vi "ExampleAsync.vi"() -> ()   [LabVIEW 2019, in "MicronTemplateAPIs.lvlib" / "MicronTemplateAPIs.lvclass"]
uses:
  MicronTemplateAPIs.lvclass
  vi.lib/Micron/gRPC/Client/Typedefs/AsyncMessageResponse.ctl
  vi.lib/Micron/gRPC/Client/Generated/MicronGRPCGeneratedClient/RPC Messages/micronGrpc_MessageRequest.ctl
  vi.lib/Micron/Base/Client/Typedefs/ServiceDetails.ctl
  78909296-a6b7-4131-b351-69347a1d12dc.vi
  9ceadd3c-745e-4cc0-becc-c9896ef65399.vi
  <vilib>/SLL Toolkit/SLL File IO/SLL File IO.lvlib
  vi.lib/Micron/Base/Client/MicronClient.lvclass
  vi.lib/Micron/gRPC/Client/Generated/MicronGRPCGeneratedClient/MicronGRPCGeneratedClient.lvlib
  vi.lib/Micron/gRPC/Client/MicronGRPCClient.lvclass
panel:
  in  "Collect Response?":bool
  out "Responses":T1[](array[typedef])
  in  "Repeat Count":i32=10
  in  "Connection Type":enum32{"Start New", "Connect Existing"}(tab)
  in  "Mode":string(combo)="Default"
  in  "Path":path
  in  "Port":i32=50051
  in  "ServiceID":string="micron-1"
  in  "UI":string(combo)="show"
  in  "Connection String":string="localhost:50051"
  out "error out":errorcluster
  in  "Command":string="Hello Micron!"
  in  "Payload":string="An Open Source Microservice Architecture on top of gRPC from https://github.com/KarthikAbiram/Micron"
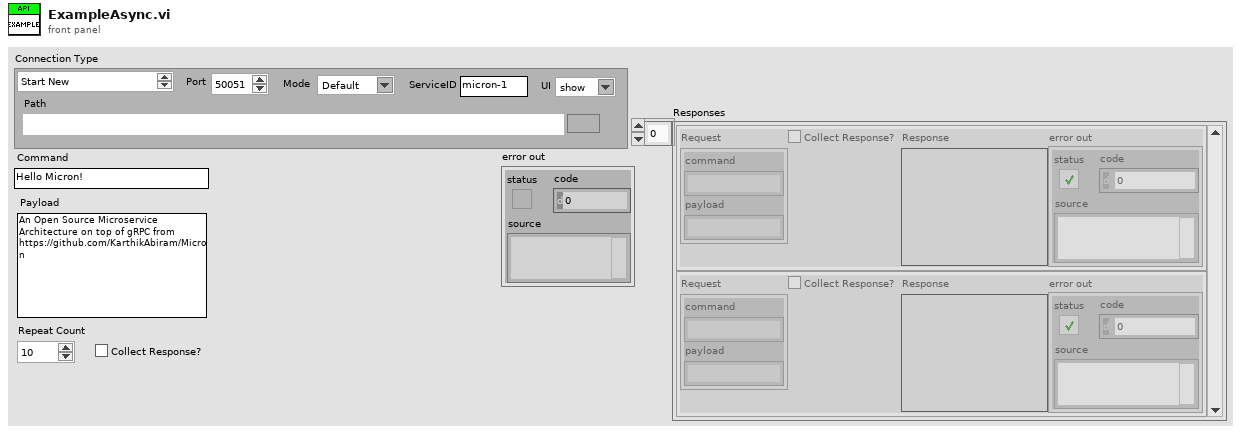
[diagram p1: front panel]
types:
  T1 = typedef "MicronGRPCClient.lvclass/AsyncMessageResponse.ctl" = cluster{"Request":T2, "Collect Response?":bool, "Response":string, "error out":errorcluster}
  T2 = typedef "MicronGRPCGeneratedClient.lvlib/micronGrpc_MessageRequest.ctl" = cluster{"command":string, "payload":string}
  T3 = typedef "MicronClient.lvclass/ServiceDetails.ctl" = cluster{"Micron Path":path, "Network":string, "ServiceID":string, "Port":i32, "FullyQualifiedName":string, "UI":string, "Args":string, "Mode":string}
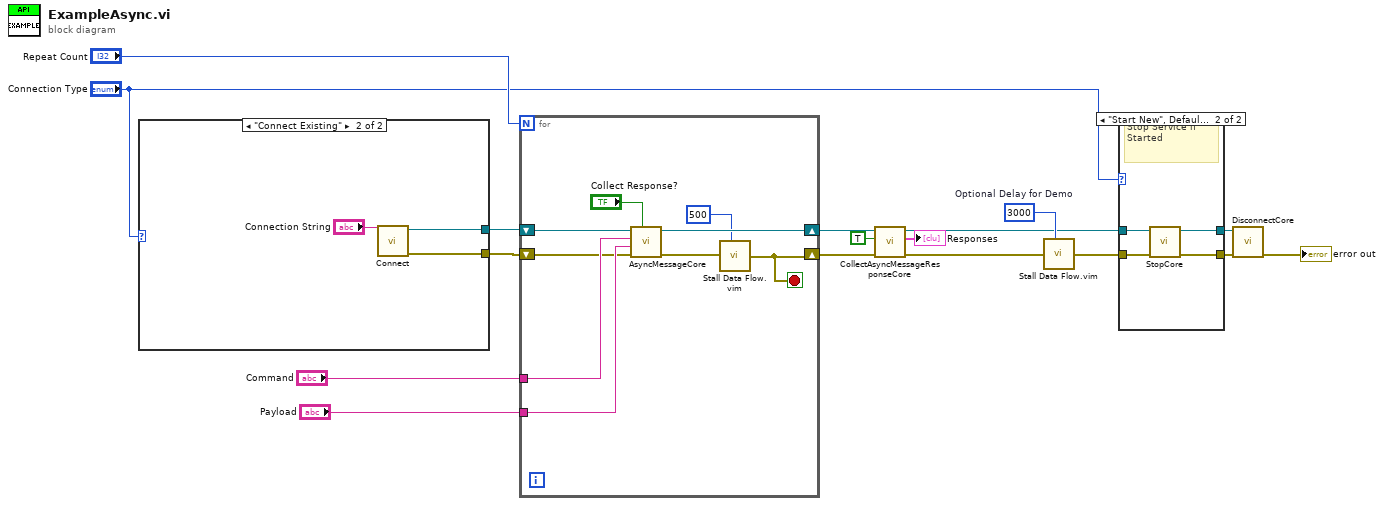
[diagram p0: block diagram]
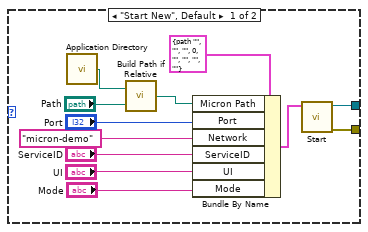
[diagram p3: hidden frame]
diagram:
  w9 = u32 3000  # Optional Delay for Demo
  n1 = case shown="\"Connect Existing\"" "Connection Type" {
    tunnel: [w29 w32] -> w14
    tunnel: [w28 w31] -> w13
    frame "Start New", Default {
      n2 = call <vilib>:"Application Directory.vi"() -> ("Application Directory"=w22:path)
      n3 = call <vilib>:"Build Path if Relative.vi"("Relative or Absolute Path"="Path", "Base Path"=w22) -> ("Path Out"=w23:path)
      n4 = Bundle By Name(cluster=T3 {"Micron Path"=path "", "Network"="", "ServiceID"="", "Port"=0, "FullyQualifiedName"="", "UI"="", "Args"="", "Mode"=""} ("Service Details"), "Micron Path"=w23, "Port"="Port", "Network"="micron-demo", "ServiceID"="ServiceID", "UI"="UI", "Mode"="Mode") -> (w26:T3)
      n5 = call "Start.vi"("Service Details"=w26) -> ("error out"=w29:errorcluster, "MicronTemplateAPIs out"=w28:refnum<class "MicronTemplateAPIs.lvclass">)  [unwired: 9 in]
    }
    frame "Connect Existing" {
      n6 = call "Connect.vi"("Connection String"="Connection String") -> ("error out"=w32:errorcluster, "MicronTemplateAPIs out"=w31:refnum<class "MicronTemplateAPIs.lvclass">)  [unwired: 9 in]
    }
  }
  n7 = for {
    N: "Repeat Count" -> [_]
    tunnel: "Payload" -> [w41]
    tunnel: "Command" -> [w40]
    shift-right: [w33] -> w7
    shift-left: w14 -> [w39]
    shift-right: [w37] -> w6
    shift-left: w13 -> [w38]
    stop <- w33 stop-if-true
    n8 = call-dynamic "AsyncMessageCore.vi"("Collect Response?"="Collect Response?", "error in (no error)"=w39, "Payload"=w41, "Command"=w40, "GRPCClient in"=w38) -> ("error out"=w36:errorcluster, "GRPCClient out"=w37:refnum<class "MicronTemplateAPIs.lvclass">)  [unwired: 5 in]
    n9 = call "Stall Data Flow.vim"("value in"=w36, "milliseconds to wait"=u32 500) -> ("value out"=w33:errorcluster)  [unwired: 1 out]
  }
  n10 = call-dynamic "CollectAsyncMessageResponseCore.vi"("error in (no error)"=w7, "Wait for All Messages?"=TRUE, "MicronGRPCClient in"=w6) -> ("error out"=w5:errorcluster, "Responses"=→"Responses":T1[], "MicronGRPCClient out"=w4:refnum<class "MicronTemplateAPIs.lvclass">)  [unwired: 6 in]
  n11 = call "Stall Data Flow.vim"("value in"=w5, "milliseconds to wait"=w9) -> ("value out"=w10:errorcluster)  [unwired: 1 out]
  n12 = case shown="\"Start New\", Default" "Connection Type" {
    tunnel: w10 -> [w43 w47]
    tunnel: w4 -> [w42 w46]
    tunnel: [w42 w45] -> w12
    tunnel: [w43 w44] -> w11
    frame "Connect Existing" {
    }
    frame "Start New", Default {
      # "Stop Service if Started"
      n13 = call-dynamic "StopCore.vi"("error in (no error)"=w47, "MicronGRPCClient in"=w46) -> ("error out"=w44:errorcluster, "MicronGRPCClient out"=w45:refnum<class "MicronTemplateAPIs.lvclass">)  [unwired: 7 in, 1 out]
    }
  }
  n14 = call-dynamic "DisconnectCore.vi"("error in (no error)"=w11, "GRPCClient in"=w12) -> ("error out"=→"error out":errorcluster)  [unwired: 8 in, 1 out]
